vi "MB Ethernet Example Slave (Legacy).vi"() -> ()   [LabVIEW 2011]
uses:
  MB Globals.vi
panel:
  in  "Listening Port":u16=502
  in  "Stop":bool
  out "Holding Registers":u16[](array[numeric]) caption="Holding Registers (Master can write in these registers)"
  out "Coils":bool[](array[boolean]) caption="Coils (Master can write coils)"
  in  "Discrete Inputs":bool[](array[boolean]) caption="Discrete Inputs (Master can only read them)"
  in  "Input Registers":u16[](array[numeric]) caption="Input Registers (Master can only read them)"
  # "MB Ethernet Example Slave.vi\n\nInstructions\n1. Run this VI first (Slave/Server)\n2. Open and run MB Ethernet Example Master.vi\n3. Modify the discrete inputs or input registers on the slave -> they're updated on the master.\n4. Modify the coils and registers on the master -> they're updated on the slave."
  # "Slave Registers"
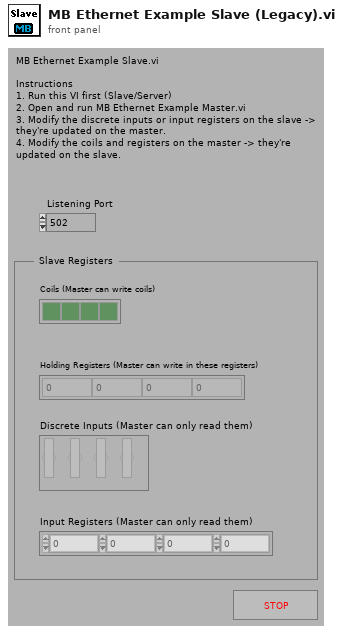
[diagram p1: front panel]
types:
  T1 = enum16{"Discrete Inputs", "Coils", "Input Registers", "Holding Registers"}
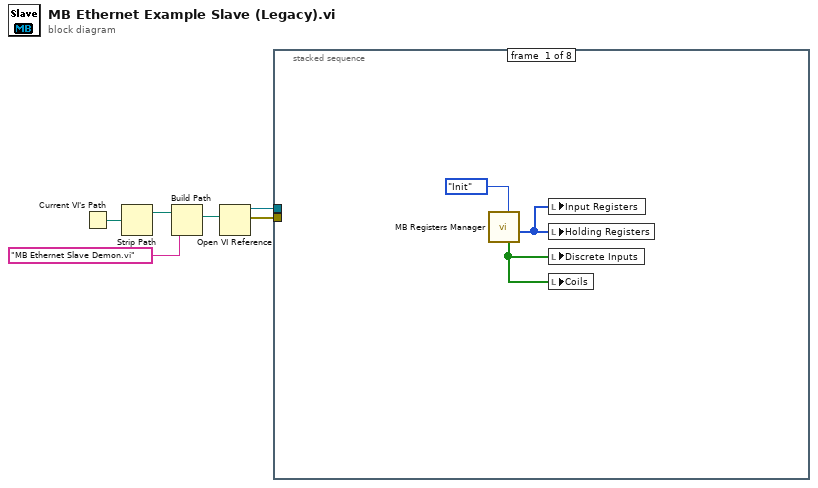
[diagram p0: block diagram]
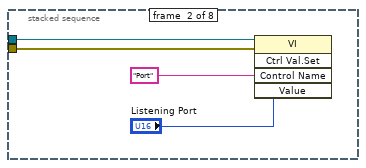
[diagram p2: hidden frame]
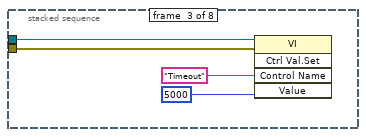
[diagram p3: hidden frame]
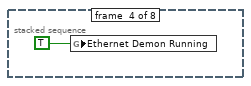
[diagram p4: hidden frame]
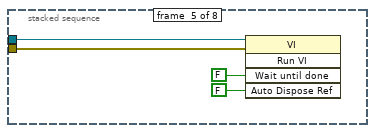
[diagram p5: hidden frame]
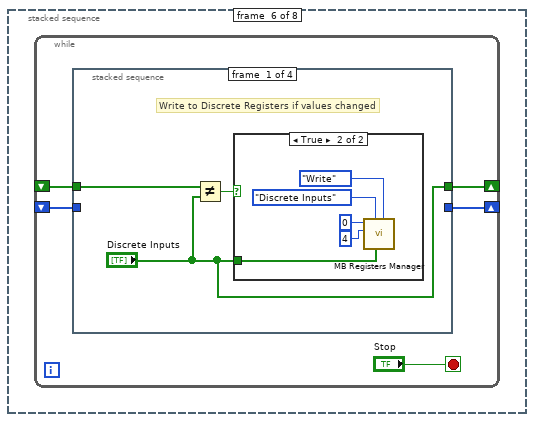
[diagram p6: hidden frame]
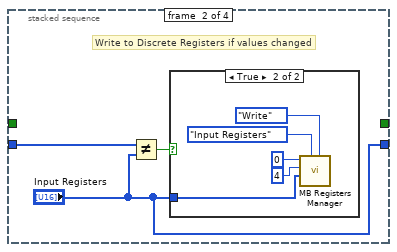
[diagram p8: hidden frame]
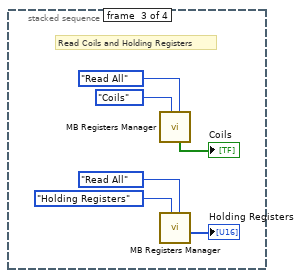
[diagram p10: hidden frame]
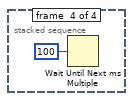
[diagram p11: hidden frame]
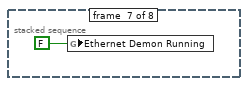
[diagram p12: hidden frame]
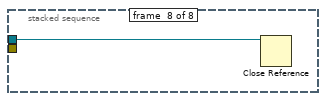
[diagram p13: hidden frame]
diagram:
  n1 = Current VI's Path() -> (path=w6:path)
  n2 = Strip Path(path=w6) -> (stripped path=w5:path)  [unwired: 1 out]
  n3 = Build Path(base path=w5, name or relative path="MB Ethernet Slave Demon.vi") -> (appended path=w3:path)
  n4 = Open VI Reference(vi path=w3) -> (vi reference=w2:refnum<vi>, error out=w1:errorcluster)  [unwired: 1 in, 4 out]
  n5 = stacked-sequence {
    tunnel: w2 -> [_ w13 w17 _ w22 _ _ w52]
    tunnel: w1 -> [_ w12 w16 _ w21 _ _ _]
    frame #0 {
      n6 = call "MB Registers Manager.vi"("Function"=enum16{"Init", "Read", "Write", "Read All"}."Init") -> ("Words out"=w8:u16[], "Bits out"=w7:bool[])  [unwired: 6 in, 3 out]
      n7 = local write "Input Registers"(w8) -> ()
      n8 = local write "Holding Registers"(w8) -> ()
      n9 = local write "Discrete Inputs"(w7) -> ()
      n10 = local write "Coils"(w7) -> ()
    }
    frame #1 {
      n11 = invoke class="VI" method="Ctrl Val.Set"(reference=w13, error in=w12, "Control Name"="Port", "Value"="Listening Port") -> ()  [unwired: 1 in, 5 out]
    }
    frame #2 {
      n12 = invoke class="VI" method="Ctrl Val.Set"(reference=w17, error in=w16, "Control Name"="Timeout", "Value"=u32 5000 ("Timeout")) -> ()  [unwired: 1 in, 5 out]
    }
    frame #3 {
      n13 = global write "MB Globals.vi" "Ethernet Demon Running"(TRUE ("Slave Demon Running")) -> ()
    }
    frame #4 {
      n14 = invoke class="VI" method="Run VI"(reference=w22, error in=w21, "Wait until done"=FALSE, "Auto Dispose Ref"=FALSE) -> ()  [unwired: 1 in, 5 out]
    }
    frame #5 {
      n15 = while {
        shift-right: [w26] -> _
        shift-left: _ -> [w25]
        shift-right: [w23] -> _
        shift-left: _ -> [w24]
        stop <- "Stop" stop-if-true
        n16 = stacked-sequence {
          tunnel: ["Discrete Inputs" _ _ _] -> w26
          tunnel: w25 -> [w30 _ _ _]
          tunnel: w24 -> [_ w37 _ _]
          tunnel: [_ "Input Registers" _ _] -> w23
          frame #0 {
            # "Write to Discrete Registers if values changed"
            n17 = Not Equal?(x=w30, y="Discrete Inputs") -> (x != y?=w28:bool)
            n18 = case shown="True" w28 {
              tunnel: "Discrete Inputs" -> [_ w31]
              frame False {
              }
              frame True {
                n19 = call "MB Registers Manager.vi"("Function"=enum16{"Init", "Read", "Write", "Read All"}."Write", "Bits In"=w31, "Table"=T1."Discrete Inputs", "Length"=u16 4, "Start Address"=u16 0) -> ()  [unwired: 2 in, 5 out]
              }
            }
          }
          frame #1 {
            # "Write to Discrete Registers if values changed"
            n20 = Not Equal?(x=w37, y="Input Registers") -> (x != y?=w38:bool)
            n21 = case shown="True" w38 {
              tunnel: "Input Registers" -> [_ w39]
              frame False {
              }
              frame True {
                n22 = call "MB Registers Manager.vi"("Function"=enum16{"Init", "Read", "Write", "Read All"}."Write", "Table"=T1."Input Registers", "Words In"=w39, "Length"=u16 4, "Start Address"=u16 0) -> ()  [unwired: 2 in, 5 out]
              }
            }
          }
          frame #2 {
            # "Read Coils and Holding Registers"
            n23 = call "MB Registers Manager.vi"("Function"=enum16{"Init", "Read", "Write", "Read All"}."Read All", "Table"=T1."Coils") -> ("Bits out"=→"Coils":bool[])  [unwired: 5 in, 4 out]
            n24 = call "MB Registers Manager.vi"("Function"=enum16{"Init", "Read", "Write", "Read All"}."Read All", "Table"=T1."Holding Registers") -> ("Words out"=→"Holding Registers":u16[])  [unwired: 5 in, 4 out]
          }
          frame #3 {
            n25 = Wait Until Next ms Multiple(millisecond multiple=u32 100) -> ()  [unwired: 1 out]
          }
        }
      }
    }
    frame #6 {
      n26 = global write "MB Globals.vi" "Ethernet Demon Running"(FALSE ("Slave Demon Running")) -> ()
    }
    frame #7 {
      n27 = Close Reference(reference=w52) -> ()  [unwired: 1 in, 1 out]
    }
  }
